vi "Apply Damage.vi"(10 "Damage":i32, 11 "Ship in":refnum<class "Ship.lvclass">) -> (3 "Ship out":refnum<class "Ship.lvclass">)   [LabVIEW 2021, in "Ship.lvclass"]
uses:
  Ship.lvclass
  C:/dev/LabVIEW/LabMelee/Source/Application Specific/Element/Element.lvclass
  Ship.lvclass/Ship.ctl
  Element/Element.lvclass/Element.ctl
  Element/Element.lvclass
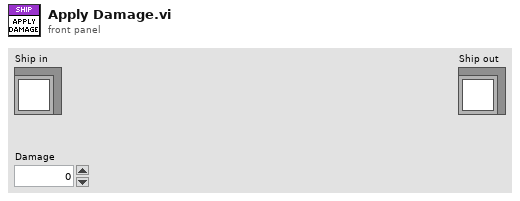
[diagram p1: front panel]
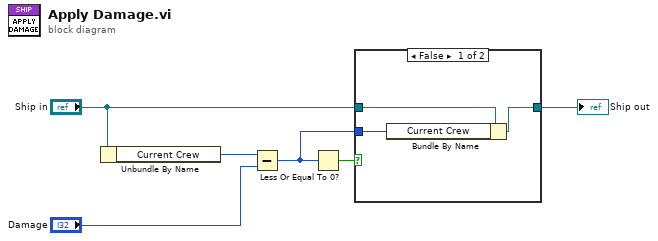
[diagram p0: block diagram]
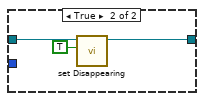
[diagram p2: hidden frame]
diagram:
  n1 = Unbundle By Name("Ship in") -> ("Current Crew"=w6:i32)
  n2 = Subtract(x=w6, y="Damage") -> (x-y=w1:i32)
  n3 = Less Or Equal To 0?(x=w1) -> (x <= 0?=w2:bool)
  n4 = case shown="False" w2 {
    tunnel: "Ship in" -> [w9 w12]
    tunnel: [w8 w11] -> w3
    tunnel: w1 -> [w7 _]
    frame False {
      n5 = Bundle By Name(cluster=w9, "Current Crew"=w7) -> (w8:refnum<class "Ship.lvclass">)
    }
    frame True {
      n6 = call "set Disappearing.vi"("Disappearing"=TRUE, "Element in"=w12) -> ("Element out"=w11:refnum<class "Ship.lvclass">)  [unwired: 9 in]
    }
  }
  "Ship out" <- w3
